vi "Calculate_Level_Triggers.vi"(11 "AllWindows":T5) -> (1 "Low0":fxp<+/-,18,5>, 2 "High0":fxp<+/-,18,5>, 3 "All_Window_Trigs":T1)   [LabVIEW 2021]
uses:
  Host/Clusts/AllWindowsClust.ctl
  Host/Clusts/ChannelWindowClust.ctl
  Controls/Clust/All_Window_Triggers_Clust.ctl
  Controls/Clust/WindowTriggerClust.ctl
  <instrlib>/_niInstr/Data Trigger/v1/Shared/Public/Level Configuration FXP(+-,18,1).ctl
  <instrlib>/_niInstr/Data Trigger/v1/Shared/Public/Level Configuration Trigger When.ctl
  <instrlib>/_niInstr/Data Trigger/v1/Shared/niInstr Data Trigger v1 Shared.lvlib
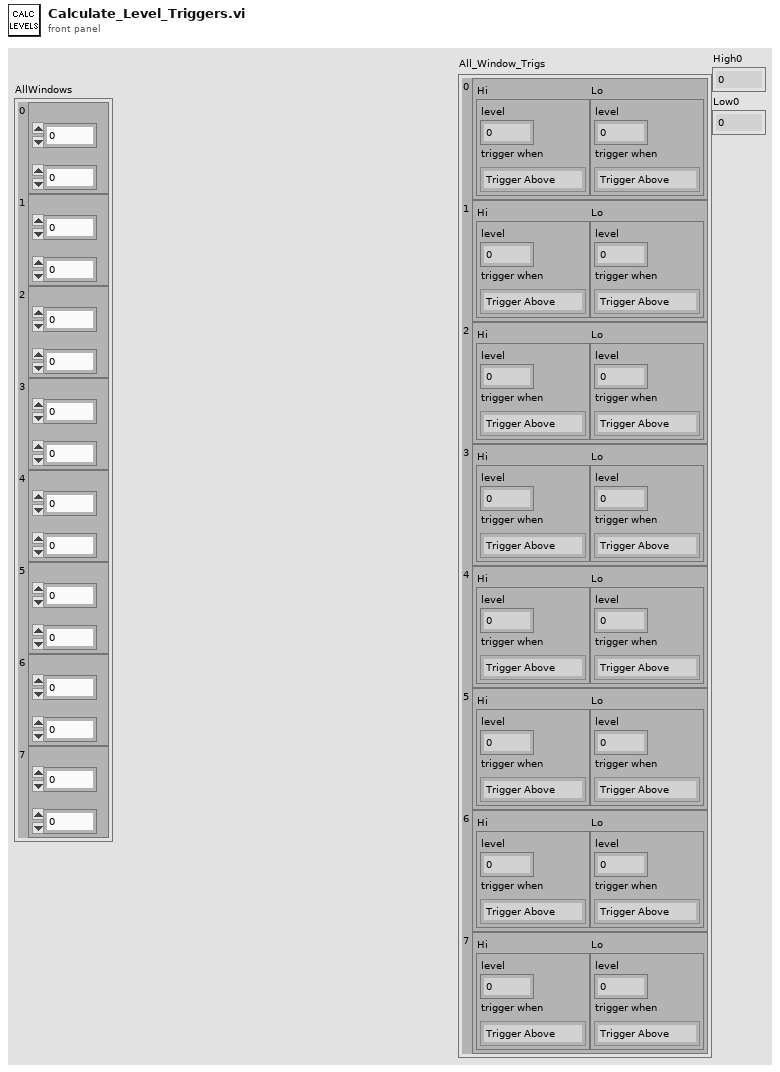
[diagram p1: front panel]
types:
  T1 = typedef "All_Window_Triggers_Clust.ctl" = cluster{"0":T2, "1":T2, "2":T2, "3":T2, "4":T2, "5":T2, "6":T2, "7":T2}
  T2 = typedef "WindowTriggerClust.ctl" = cluster{"Hi":T3, "Lo":T3}
  T3 = typedef "niInstr Data Trigger v1 Shared.lvlib/Level Configuration FXP(+-,18,1).ctl" = cluster{"level":fxp<+/-,18,5>, "trigger when":T4}
  T4 = typedef "niInstr Data Trigger v1 Shared.lvlib/Level Configuration Trigger When.ctl" = enum8{"Trigger Above", "Trigger Below"}
  T5 = typedef "AllWindowsClust.ctl" = cluster{"0":T6, "1":T6, "2":T6, "3":T6, "4":T6, "5":T6, "6":T6, "7":T6}
  T6 = typedef "ChannelWindowClust.ctl" = cluster{"HalfRange":fxp<+/-,18,5>, "StartCenter":fxp<+/-,18,5>}
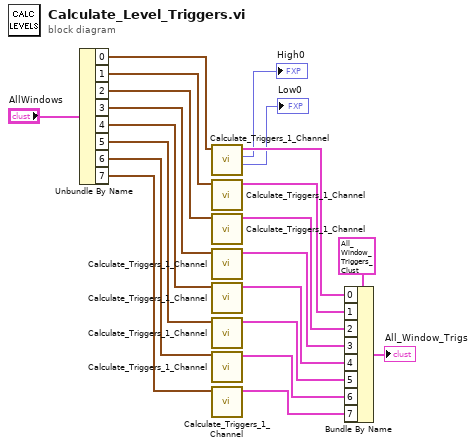
[diagram p0: block diagram]
diagram:
  n1 = Unbundle By Name("AllWindows") -> ("0"=w21:T6, "1"=w16:T6, "2"=w15:T6, "3"=w14:T6, "4"=w13:T6, "5"=w12:T6, "6"=w11:T6, "7"=w10:T6)
  n2 = call "Calculate_Triggers_1_Channel.vi"("ChanSettings"=w21) -> ("Low"=→"Low0":fxp<+/-,18,5>, "High"=→"High0":fxp<+/-,18,5>, "WindowTrig"=w17:T2)  [unwired: 8 in]
  n3 = call "Calculate_Triggers_1_Channel.vi"("ChanSettings"=w16) -> ("WindowTrig"=w9:T2)  [unwired: 8 in, 2 out]
  n4 = call "Calculate_Triggers_1_Channel.vi"("ChanSettings"=w15) -> ("WindowTrig"=w8:T2)  [unwired: 8 in, 2 out]
  n5 = call "Calculate_Triggers_1_Channel.vi"("ChanSettings"=w14) -> ("WindowTrig"=w7:T2)  [unwired: 8 in, 2 out]
  n6 = call "Calculate_Triggers_1_Channel.vi"("ChanSettings"=w13) -> ("WindowTrig"=w6:T2)  [unwired: 8 in, 2 out]
  n7 = call "Calculate_Triggers_1_Channel.vi"("ChanSettings"=w12) -> ("WindowTrig"=w5:T2)  [unwired: 8 in, 2 out]
  n8 = call "Calculate_Triggers_1_Channel.vi"("ChanSettings"=w11) -> ("WindowTrig"=w4:T2)  [unwired: 8 in, 2 out]
  n9 = call "Calculate_Triggers_1_Channel.vi"("ChanSettings"=w10) -> ("WindowTrig"=w3:T2)  [unwired: 8 in, 2 out]
  n10 = Bundle By Name(cluster=T1 {"0"={"Hi"={"level"=0.0, "trigger when"=enum."Trigger Above"}, "Lo"={"level"=0.0, "trigger when"=enum."Trigger Below"}}, "1"={"Hi"={"level"=0.0, "trigger when"=enum."Trigger Above"}, "Lo"={"level"=0.0, "trigger when"=enum."Trigger Below"}}, "2"={"Hi"={"level"=0.0, "trigger when"=enum."Trigger Above"}, "Lo"={"level"=0.0, "trigger when"=enum."Trigger Below"}}, "3"={"Hi"={"level"=0.0, "trigger when"=enum."Trigger Above"}, "Lo"={"level"=0.0, "trigger when"=enum."Trigger Below"}}, "4"={"Hi"={"level"=0.0, "trigger when"=enum."Trigger Above"}, "Lo"={"level"=0.0, "trigger when"=enum."Trigger Below"}}, "5"={"Hi"={"level"=0.0, "trigger when"=enum."Trigger Above"}, "Lo"={"level"=0.0, "trigger when"=enum."Trigger Below"}}, "6"={"Hi"={"level"=0.0, "trigger when"=enum."Trigger Above"}, "Lo"={"level"=0.0, "trigger when"=enum."Trigger Below"}}, "7"={"Hi"={"level"=0.0, "trigger when"=enum."Trigger Above"}, "Lo"={"level"=0.0, "trigger when"=enum."Trigger Below"}}} ("All_Window_Trigs"), "0"=w17, "1"=w9, "2"=w8, "3"=w7, "4"=w6, "5"=w5, "6"=w4, "7"=w3) -> (→"All_Window_Trigs":T1)
